vi "RT_main.vi"() -> ()   [LabVIEW 2016]
uses:
  <vilib>/Platform/TimedLoop/XDataNode/timing_clust.ctl
  <vilib>/Platform/TimedLoop/XDataNode/nitl_modes.ctl
  <vilib>/Platform/TimedLoop/XDataNode/wakeup.ctl
  <vilib>/myRIO/Common/Instrument Driver Framework/myRIO v1.0/UART/vis/myRIO v1.0 Close UART.vi
  <vilib>/FPGAPlugInAG/myRIO-1900/niLvFpga_Open_myRIO-1900.vi
  <vilib>/rvi/interface/common/dynamic/niFpgaDynamicAddResources.vi
  <vilib>/Utility/error.llb/Error Cluster From Error Code.vi
  <vilib>/rvi/errors/niLvFpgaAdjustHostInterfaceError.vi
  <vilib>/myRIO/Common/Instrument Driver Framework/Utilities/vis/FPGA Ref Manager.vi
  <vilib>/myRIO/Common/Instrument Driver Framework/myRIO v1.0/myRIO v1.0 Reset FPGA.vi
  <vilib>/myRIO/Common/Instrument Driver Framework/myRIO v1.0/IRQ/vis/myRIO v1.0 IRQ Info FGV.vi
  <vilib>/myRIO/Common/Instrument Driver Framework/myRIO v1.0/IRQ/vis/myRIO v1.0 Timer IRQ Info FGV.vi
  <vilib>/myRIO/Common/Instrument Driver Framework/myRIO v1.0/IRQ/vis/myRIO v1.0 ISR Agent.vi
  <vilib>/rvi/interface/nirviOpenFPGA/nirviOpenFPGA.xnode
  FPGA Bitfiles/CraneProject_FPGATarget_MotorandEncoder(_xX61osqV1qk.lvbitx
  <vilib>/rvi/interface/nirviReadWriteControl/nirviReadWriteControl.xnode
  <vilib>/Platform/TimedLoop/XDataNode/XDataNode.xnode
  <vilib>/rvi/interface/Simulation/niFpgaSimulationCallBeginRW.vi
  <vilib>/myRIO/Instrument Drivers/Utilities/Utilities.lvlib
  NiFpgaLv.dll
  <vilib>/Platform/TimedLoop/XDataNode/XDNodeRunTimeDep.lvlib
panel:
  in  "K5":dbl
  out "degrees":dbl
  out "meters":dbl
  in  "N":dbl
  in  "K4":dbl
  in  "K3":dbl
  in  "K2":dbl
  in  "K1":dbl
  in  "HALT":bool
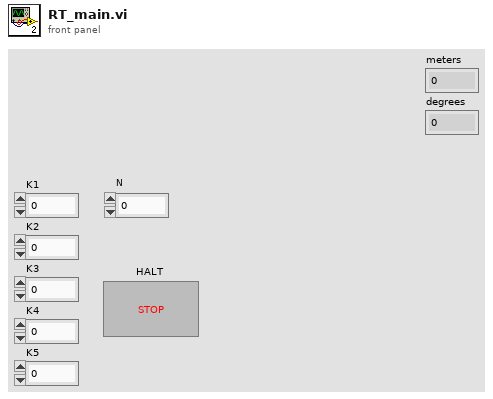
[diagram p1: front panel]
types:
  T1 = typedef "XDNodeRunTimeDep.lvlib/timing_clust.ctl" = cluster{"Expected End [f-1]":u64, "Actual End [f-1]":u64, "Finished Late? [f-1]":bool, "Expected End [i-1]":u64, "Actual End [i-1]":u64, "Finished Late? [i-1]":bool, "Expected Start [i]":u64, "Actual Start [i]":u64, "Expected Start [f]":u64, "Actual Start [f]":u64, "Source Name":string, "Structure Name":string, "Period":i64, "Deadline":i64, "Offset":i64, "Start":i64, "Priority":i32, "Timeout":i32, "Mode":T2, "Wakeup Reason":T3, "Error":errorcluster, "Source Type":string, "Secondary Source Type":string, "Global End Time":u64, "Global Start Time":u64, "Frame Duration":u64, "Iteration Duration":u64, "Assigned CPU":i32, "I/O Scan Engine Mode":u32}
  T2 = typedef "XDNodeRunTimeDep.lvlib/nitl_modes.ctl" = enum32{"No Change", "Process missed periods, maintain original phase", "Discard missed periods, maintain original phase", "Process missed periods, ignore original phase", "Discard missed periods, ignore original phase"}
  T3 = typedef "XDNodeRunTimeDep.lvlib/wakeup.ctl" = enum32{"Normal", "Aborted", "Asynchronous wakeup", "Timing source error", "Timed loop error", "Timeout"}
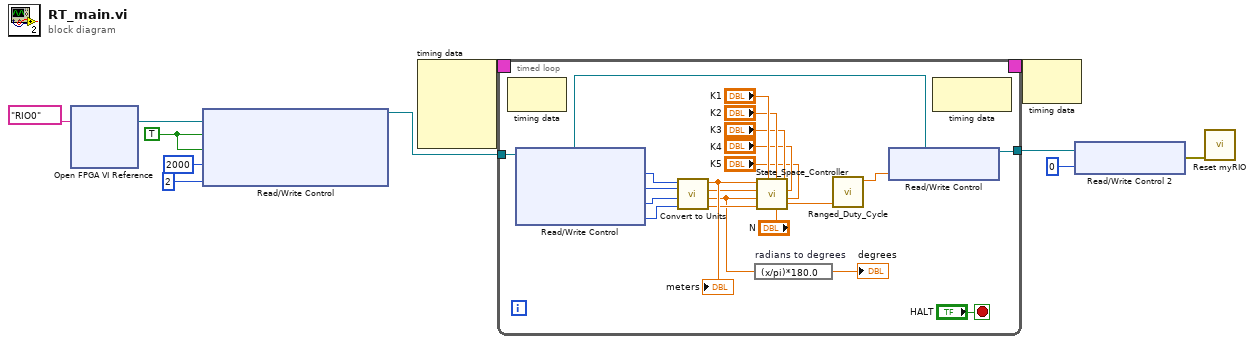
[diagram p0: block diagram]
diagram:
  w9 = TRUE ("Reset Encoder Position")
  n1 = xnode "Open FPGA VI Reference"("resource name"=tag "RIO0") -> ("FPGA VI Reference Out"=w11:refnum<k20>)  [unwired: 1 in, 1 out]
  n2 = xnode "Read/Write Control"("FPGA VI Reference In"=w11, "Reset Cart Encoder Position"=w9, "Reset Fulcrum Encoder Position"=w9, "Duty Cycle Divisor"=i16 2000, "Cycles to Filter"=u16 2) -> ("FPGA VI Reference Out"=w4:refnum<k20>)  [unwired: 1 in, 1 out]
  n3 = node-c288() -> (w6:T1)  [unwired: 4 in]
  n4 = timed-loop {
    timing: w6 -> [_]
    timing-out: [_] -> w5
    tunnel: w4 -> [w32]
    tunnel: [w31] -> w3
    stop <- "HALT" stop-if-true
    n5 = node-c288() -> ()  [unwired: 1 in, 1 out]
    n6 = xnode "Read/Write Control"("FPGA VI Reference In"=w32) -> ("FPGA VI Reference Out"=w30:refnum<k20>, "Cart Position"=w16:i32, "Cart Period Ticks"=w28:i32, "Fulcrum Position"=w15:i32, "Fulcrum Period Ticks"=w27:i32)  [unwired: 1 in, 1 out]
    n7 = call "Convert to Units.vi"("Fulcrum Ticks"=w27, "Fulcrum Counts"=w15, "Cart Ticks"=w28, "Cart Counts"=w16) -> ("rad/sec"=w24:dbl, "rad"=w14:dbl, "meters/sec"=w25:dbl, "meters"=w26:dbl)  [unwired: 4 in]
    "meters" <- w26
    n8 = expression code="(x/pi)*180.0" "radians to degrees"(w14) -> (→"degrees":dbl)
    n9 = call "State_Space_Controller.vi"("K5"="K5", "K4"="K4", "K3"="K3", "N"="N", "K2"="K2", "K1"="K1", "Rads/Sec"=w24, "Rads"=w14, "Meters/Sec"=w25, "Meters"=w26) -> ("output"=w18:dbl)  [unwired: 1 in]
    n10 = call "Ranged_Duty_Cycle.vi"("Volt Input"=w18) -> ("Duty Cycle"=w17:dbl)  [unwired: 10 in]
    n11 = xnode "Read/Write Control"("FPGA VI Reference In"=w30, "Duty Cycle (ticks)"=w17) -> ("FPGA VI Reference Out"=w31:refnum<k20>)  [unwired: 1 in, 1 out]
    n12 = node-c288() -> ()  [unwired: 1 in, 1 out]
  }
  n13 = node-c288(w5) -> ()  [unwired: 1 out]
  n14 = xnode ("Read/Write Control 2")("FPGA VI Reference In"=w3, "Duty Cycle (ticks)"=i16 0) -> ("error out"=w1:errorcluster)  [unwired: 1 in, 1 out]
  n15 = call <vilib>:"Reset myRIO.vi"("error in (no error)"=w1) -> ()  [unwired: 10 in, 1 out]
